vi "MA-DAQ_house_debugOnly.vi"() -> ()   [LabVIEW 2014]
panel:
  out "Running":bool
  out "P1":T1
  out "P0":T2
  out "error out":errorcluster
  out "?":bool
  out "?":bool
  out "?":bool
  out "?":bool
  out "?":bool
  out "?":bool
  out "?":bool
  out "?":bool
  out "?":bool
  out "?":bool
  out "8 wire data":u8
  in  "DAC  1 [V]":dbl min=0.0 max=2.0
  in  "VISA resource name":refnum<visa-resource-name>
  out "Device ID":string
  in  "Stop Button":bool
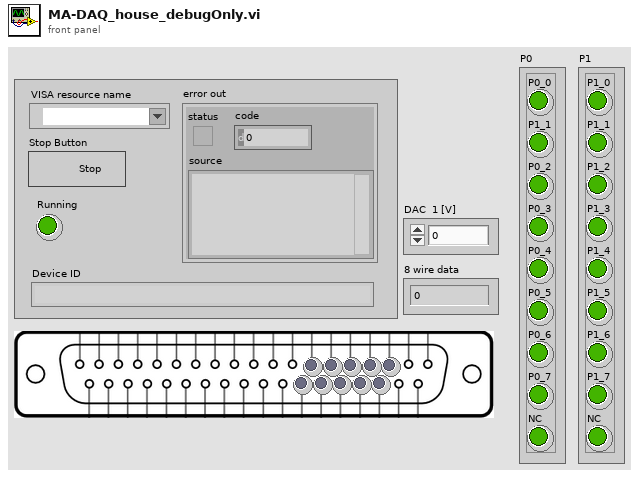
[diagram p1: front panel]
types:
  T1 = cluster{"P1_0":bool, "P1_1":bool, "P1_2":bool, "P1_3":bool, "P1_4":bool, "P1_5":bool, "P1_6":bool, "P1_7":bool, "NC":bool}
  T2 = cluster{"P0_0":bool, "P1_1":bool, "P0_2":bool, "P0_3":bool, "P0_4":bool, "P0_5":bool, "P0_6":bool, "P0_7":bool, "NC":bool}
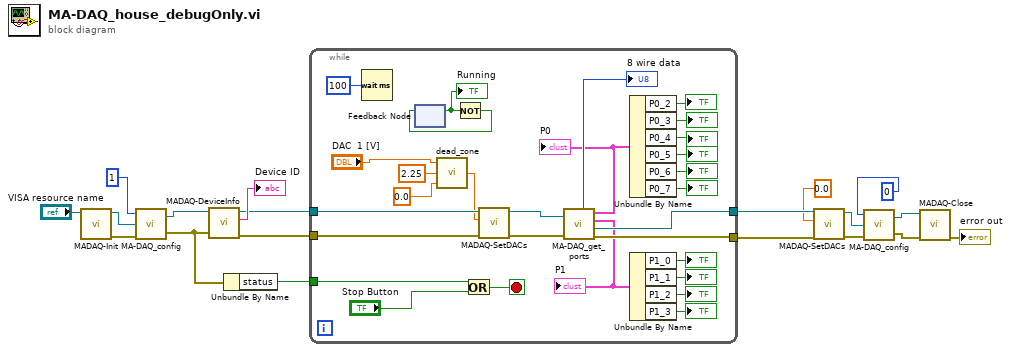
[diagram p0: block diagram]
diagram:
  n1 = call "MADAQ-Init.vi"("VISA resource name"="VISA resource name") -> ("error out"=w9:errorcluster, "VISA resource name out"=w10:refnum<visa-resource-name>)  [unwired: 5 in]
  n2 = call "MA-DAQ_config.vi"("error in (no error)"=w9, "VISA Refnum in"=w10, "mode"=u8 1) -> ("error out"=w7:errorcluster, "VISA Refnum out"=w8:refnum<visa-resource-name>)
  n3 = call "MADAQ-DeviceInfo.vi"("error in (no error)"=w7, "VISA resource name"=w8) -> ("error out"=w18:errorcluster, "Device ID"=→"Device ID":string, "VISA resource name out"=w16:refnum<visa-resource-name>)  [unwired: 3 in]
  n4 = Unbundle By Name(w7) -> ("status"=w12:bool)
  n5 = while {
    tunnel: w18 -> [w47]
    tunnel: w16 -> [w46]
    tunnel: [w39] -> w14
    tunnel: [w43] -> w15
    tunnel: w12 -> [w41]
    stop <- w42 stop-if-true
    n6 = Wait (ms)(milliseconds to wait=u32 100) -> ()  [unwired: 1 out]
    n7 = feedback #1() -> (w21:bool)  [unwired: 1 in]
    "Running" <- w21
    n8 = call "dead_zone.vi"("min"=0.0, "max"=2.25, "number in"="DAC  1 [V]") -> ("number out"=w25:dbl)
    n9 = Not(x=w21) -> (.not. x?=w20:bool)
    n10 = feedback-in #1(w20) -> ()
    n11 = Or(x=w41, y="Stop Button") -> (x .or. y?=w42:bool)
    n12 = call "MADAQ-SetDACs.vi"("error in (no error)"=w47, "DAC  1 [V]"=w25, "VISA resource name"=w46) -> ("error out"=w44:errorcluster, "VISA resource name out"=w45:refnum<visa-resource-name>)  [unwired: 3 in]
    n13 = call "MA-DAQ_get_ports.vi"("error in (no error)"=w44, "VISA Refnum in"=w45) -> ("error out"=w43:errorcluster, "VISA Refnum out"=w39:refnum<visa-resource-name>, "P1"=w37:T1, "P0"=w32:T2, "data"=→"8 wire data":u8)
    "P0" <- w32
    "P1" <- w37
    n14 = Unbundle By Name(w32) -> ("P0_2"=→"?":bool, "P0_3"=→"?":bool, "P0_4"=→"?":bool, "P0_5"=→"?":bool, "P0_6"=→"?":bool, "P0_7"=→"?":bool)
    n15 = Unbundle By Name(w37) -> ("P1_0"=→"?":bool, "P1_1"=→"?":bool, "P1_2"=→"?":bool, "P1_3"=→"?":bool)
  }
  n16 = call "MADAQ-SetDACs.vi"("error in (no error)"=w15, "DAC  1 [V]"=0.0, "VISA resource name"=w14) -> ("error out"=w4:errorcluster, "VISA resource name out"=w5:refnum<visa-resource-name>)  [unwired: 3 in]
  n17 = call "MA-DAQ_config.vi"("error in (no error)"=w4, "VISA Refnum in"=w5, "mode"=u8 0) -> ("error out"=w3:errorcluster, "VISA Refnum out"=w2:refnum<visa-resource-name>)
  n18 = call "MADAQ-Close.vi"("error in (no error)"=w3, "VISA resource name"=w2) -> ("error out"=→"error out":errorcluster)  [unwired: 4 in, 1 out]
